vi "ConfigureFLIRAX5.vi"(8 "error in (no error)":errorcluster, 10 "IR camera settings":T1={"emissitivity"=0.99, "reflected temperature"=273.15, "window transmission"=0.99, "window temperature"=273.15, "atmospheric transmission"=0.99, "atmospheric temperature"=273.15}, 11 "IMAQdx Session":T2) -> (0 "error out":errorcluster, 3 "IMAQdx Session out":T2)   [LabVIEW 2017, in "IrAcquisition.lvlib"]
uses:
  <vilib>/addons/InsightCM/Devices/Shared/Ir/IrAcquisition/IrAcquisition.lvlib
  <vilib>/userdefined/High Color/IMAQdx.ctl
  <vilib>/addons/InsightCM/Devices/Shared/Ir/IrAcquisition/controls/IRCameraSettings.ctl
  <resource>/objmgr/imaqdx.rc
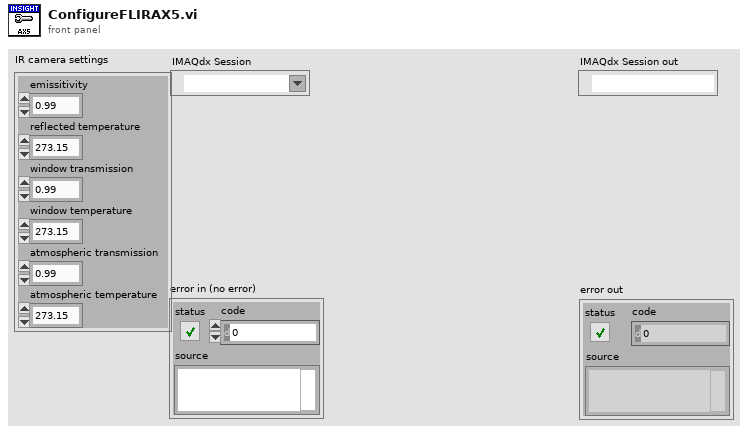
[diagram p1: front panel]
types:
  T1 = typedef "IrAcquisition.lvlib/IRCameraSettings.ctl" = cluster{"emissitivity":dbl, "reflected temperature":dbl, "window transmission":dbl, "window temperature":dbl, "atmospheric transmission":dbl, "atmospheric temperature":dbl}
  T2 = typedef "IMAQdx.ctl" = refnum<k21>
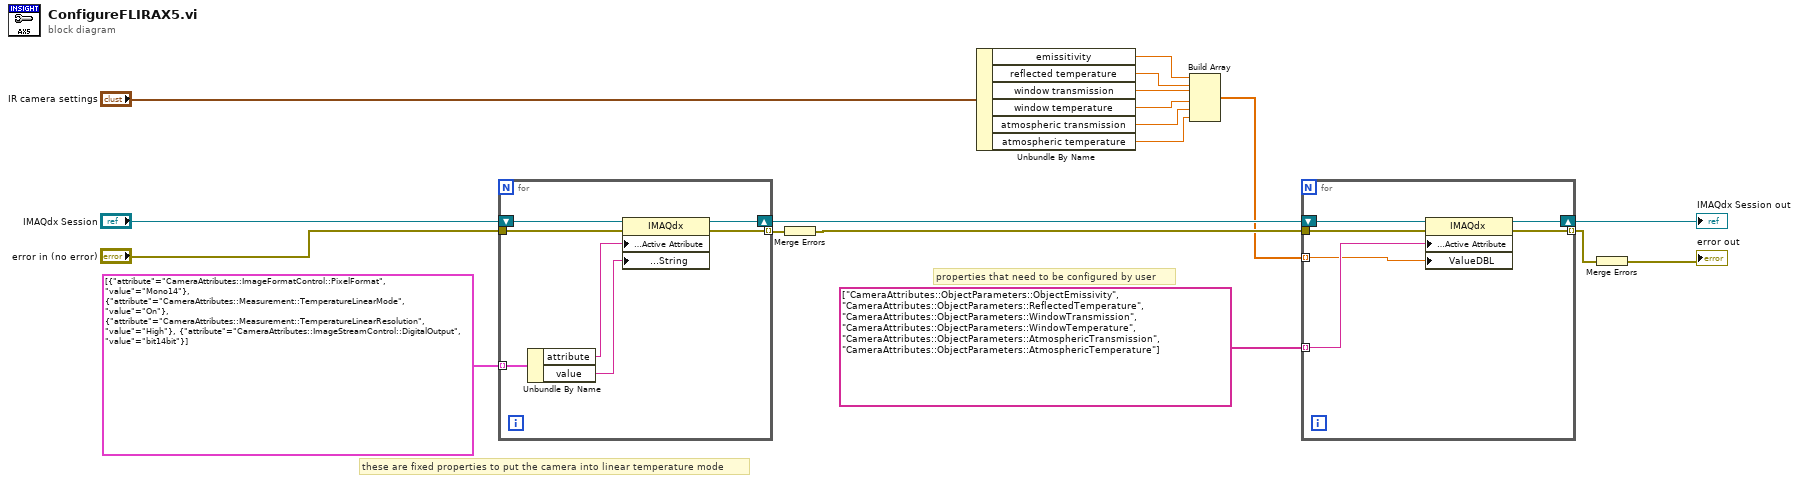
[diagram p0: block diagram]
diagram:
  # "properties that need to be configured by user"
  # "these are fixed properties to put the camera into linear temperature mode"
  n1 = for {
    tunnel: cluster{"attribute":string, "value":string}[] [{"attribute"="CameraAttributes::ImageFormatControl::PixelFormat", "value"="Mono14"}, {"attribute"="CameraAttributes::Measurement::TemperatureLinearMode", "value"="On"}, {"attribute"="CameraAttributes::Measurement::TemperatureLinearResolution", "value"="High"}, {"attribute"="CameraAttributes::ImageStreamControl::DigitalOutput", "value"="bit14bit"}] -> [w24] mode=indexing
    shift-right: [w22] -> w14
    shift-left: "IMAQdx Session" -> [w25]
    tunnel: "error in (no error)" -> [w21]
    tunnel: [w19] -> w15 mode=indexing
    n2 = Unbundle By Name(w24) -> ("attribute"=w23:string, "value"=w20:string)
    n3 = property class="IMAQdx"(reference=w25, error in=w21, "Camera Attributes:Active Attribute"=w23, "Camera Attributes:Value:String"=w20) -> (reference out=w22:T2, error out=w19:errorcluster)
  }
  n4 = Merge Errors(w15) -> (w13:errorcluster)
  n5 = Unbundle By Name("IR camera settings") -> ("emissitivity"=w7:dbl, "reflected temperature"=w6:dbl, "window transmission"=w5:dbl, "window temperature"=w4:dbl, "atmospheric transmission"=w3:dbl, "atmospheric temperature"=w2:dbl)
  n6 = Build Array(w7, w6, w5, w4, w3, w2) -> (w1:dbl[])
  n7 = for {
    shift-right: [w30] -> w10
    shift-left: w14 -> [w31]
    tunnel: w13 -> [w29]
    tunnel: [w28] -> w12 mode=indexing
    tunnel: string[] ["CameraAttributes::ObjectParameters::ObjectEmissivity", "CameraAttributes::ObjectParameters::ReflectedTemperature", "CameraAttributes::ObjectParameters::WindowTransmission", "CameraAttributes::ObjectParameters::WindowTemperature", "CameraAttributes::ObjectParameters::AtmosphericTransmission", "CameraAttributes::ObjectParameters::AtmosphericTemperature"] -> [w27] mode=indexing
    tunnel: w1 -> [w26] mode=indexing
    n8 = property class="IMAQdx"(reference=w31, error in=w29, "Camera Attributes:Active Attribute"=w27, "ValueDBL"=w26) -> (reference out=w30:T2, error out=w28:errorcluster)
  }
  "IMAQdx Session out" <- w10
  n9 = Merge Errors(w12) -> (→"error out":errorcluster)
